vi "grabber_raps.vi"() -> ()   [LabVIEW 2010]
uses:
  command_enum.ctl
  status_enum.ctl
  FPGAWrapperMH120124RAPS_PXI7813R/settings_cluster_raps.ctl
  common_typedefs/channels_cluster.ctl
  fpgaVIsAndControls/gate_cluster.ctl
  common_typedefs/gate_parameters_cluster.ctl
  motion_correction_cluster.ctl
  gui_refs.ctl
  <vilib>/rvi/interface/nirviReadWriteControl/nirviReadWriteControl.xnode
  FPGA_raps_reference.ctl
  <vilib>/rvi/interface/common/niFpgaNodeNameForErrorReporting.ctl
  <vilib>/rvi/errors/niLvFpgaWhatHappensToTopLevelVI.ctl
  <vilib>/dex/Flush And Wait Empty Condition.ctl
  <vilib>/rvi/interface/nirviMethod/nirviMethod.xnode
  <vilib>/rvi/interface/nirviCloseFPGA/nirviCloseFPGA.xnode
  <vilib>/Utility/error.llb/Error Cluster From Error Code.vi
  <vilib>/rvi/errors/niLvFpgaAdjustHostInterfaceError.vi
  <vilib>/FPGAPlugInAG/Dynamic/niLvFpga_Close_Dynamic.vi
  NiFpgaLv.dll
panel:
  out "offset (y,x)":i16[](array[numeric])
  in  "total amount pixels":i32
  in  "channel":i8
  in  "# square points":i32
  in  "reference array":u16[][](graph)
  out "data out":T1={"number of pixels"=0, "point package size"=0, "maximum bit-depth"=0, "AOD amplitude"=0, "pixel dwell time"=0.0, "ra trajectory pixels (data/pixels transfered)"=0, "channel offsets"={"channel 0"=0, "channel 1"=0, "channel 2"=0, "channel 3"=0}, "offset (Hz)"=[], "RAPS array"=[], "gates"=[], "enable clocks?"=-1, "motion correction"={"reference array"=[], "# square points"=0, "channel"=0}}
  in  "first pixel is zero?":bool caption="first pixel is zero? (set to TRUE for debugging only)"
  out "current pixel no.":i64
  out "read size":u32
  out "Elements Remaining":u32
  out "stop":bool
  out "current status":T5
  out "pixel no.":i64
  out "last command_not_acq":T6
  out "FIFO overflow?":bool
  out "last command?":T6
  out "error out":errorcluster
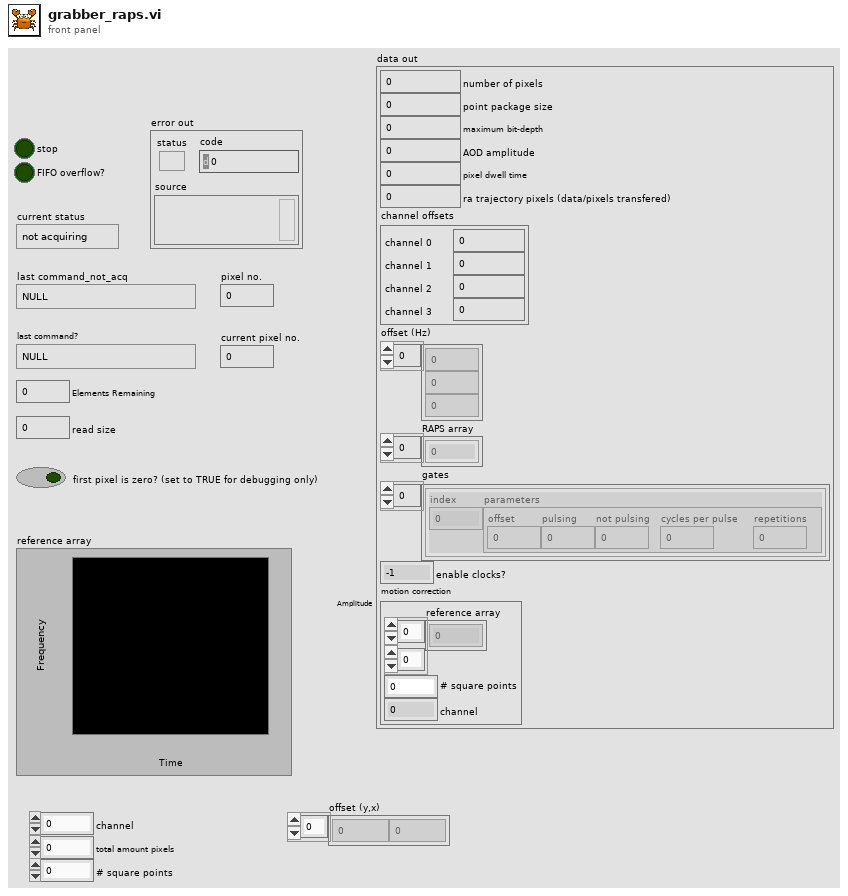
[diagram p1: front panel]
types:
  T1 = typedef "settings_cluster_raps.ctl" = cluster{"number of pixels":i64, "point package size":u8, "maximum bit-depth":i8, "AOD amplitude":u16, "pixel dwell time":dbl, "ra trajectory pixels (data/pixels transfered)":u32, "channel offsets":T2, "offset (Hz)":dbl[], "RAPS array":u64[], "gates":T3[], "enable clocks?":i16, "motion correction":cluster{"reference array":u16[][], "# square points":i32, "channel":i8}}
  T2 = typedef "channels_cluster.ctl" = cluster{"channel 0":u32, "channel 1":u32, "channel 2":u32, "channel 3":u32}
  T3 = typedef "gate_cluster.ctl" = cluster{"index":i32, "parameters":T4}
  T4 = typedef "gate_parameters_cluster.ctl" = cluster{"offset":i64, "pulsing":i64, "not pulsing":i64, "cycles per pulse":i64, "repetitions":i64}
  T5 = typedef "status_enum.ctl" = enum16{"not acquiring", "acquiring"}
  T6 = typedef "command_enum.ctl" = enum8{"NULL", "update", "start", "stop", "reset", "shut-down"}
  T7 = typedef "gui_refs.ctl" = cluster{"reference array":refnum<vi>, "total amount pixels":refnum<vi>, "# square points":refnum<vi>, "channel":refnum<vi>}
  T8 = typedef "motion_correction_cluster.ctl" = cluster{"reception":cluster{"square length":i32, "offset":i32, "# squares out":i32, "left over":u16[], "raps points length":i32}, "fft":cluster{"reference":dbl[][]}}
  T9 = typedef "FPGA_raps_reference.ctl" = refnum<k20>
  T10 = typedef "network_streaming_queues_cluster.ctl" = cluster{"command reader":refnum<k21>, "data writer":refnum<k21>, "raps reader":refnum<k21>, "settings framescan reader":refnum<k21>, "configuration framescan reader":refnum<k21>, "settings raps reader":refnum<k21>, "configuration raps reader":refnum<k21>, "update queue":refnum<queue>}
  T11 = typedef "niFpgaNodeNameForErrorReporting.ctl" = enum16{"Open FPGA VI Reference", "Read/Write Control", "Invoke Method: Abort", "Invoke Method: Acknowledge IRQ", "Invoke Method: Download", "Invoke Method: FIFO.Configure", "Invoke Method: FIFO.Read", "Invoke Method: FIFO.Start", "Invoke Method: FIFO.Stop", "Invoke Method: FIFO.Write", "Invoke Method: Reset", "Invoke Method: Run", "Invoke Method: Wait on IRQ", "Close FPGA VI Reference"}
  T12 = typedef "niLvFpgaWhatHappensToTopLevelVI.ctl" = enum16{"top level VI scripted behind XNode", "top level VI inlined behind XNode"}
  T13 = typedef "Flush And Wait Empty Condition.ctl" = u8
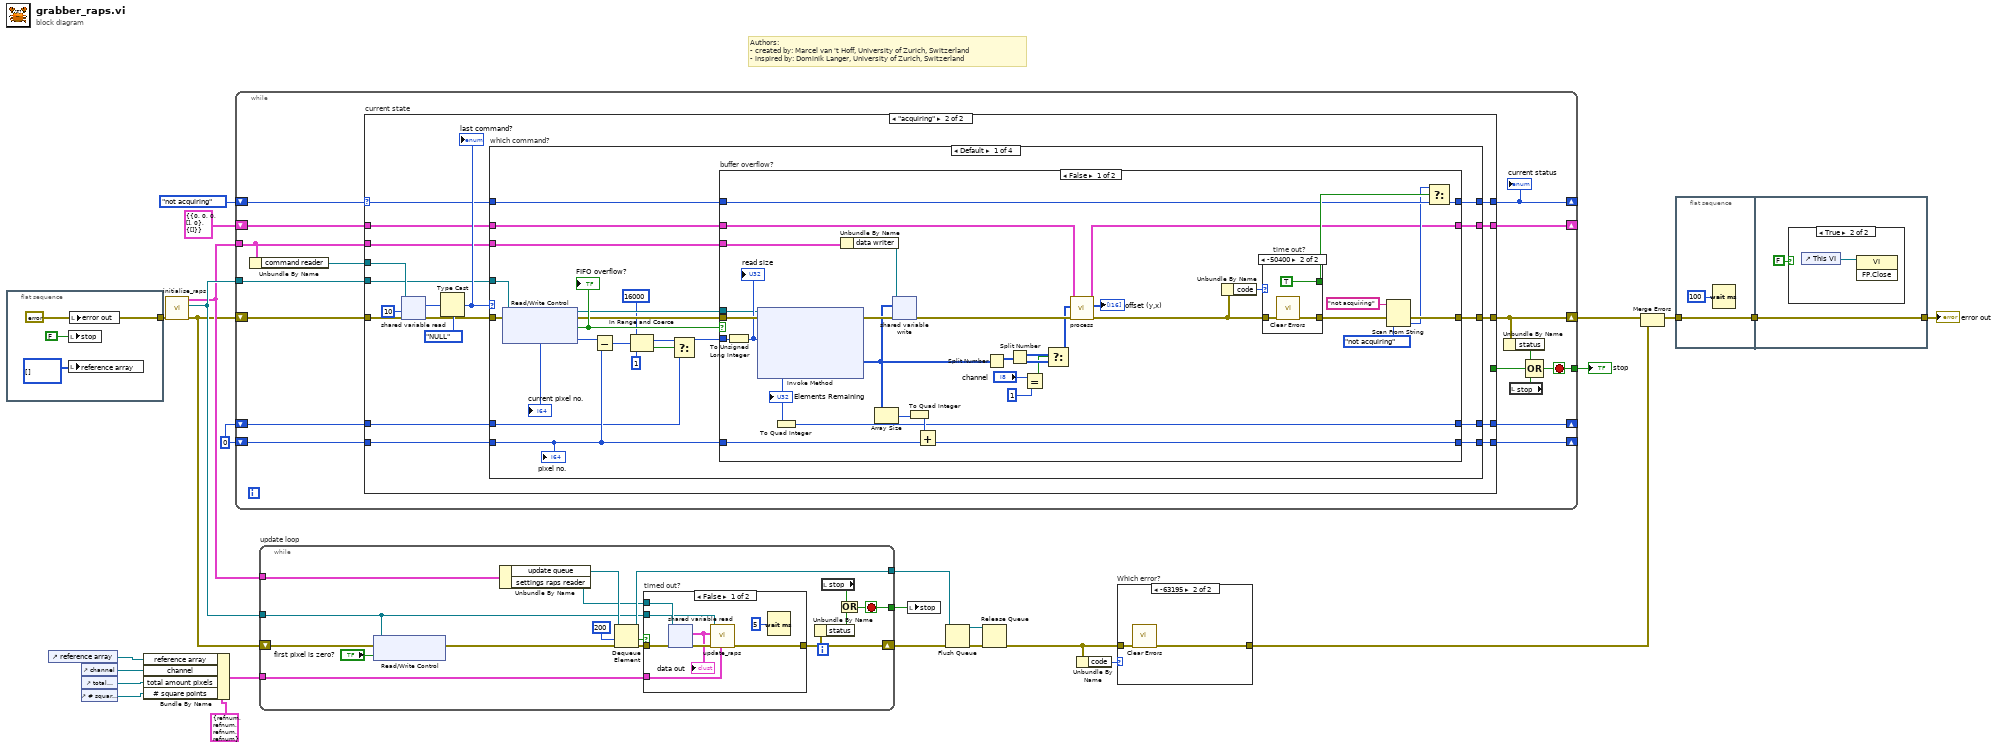
[diagram p0: block diagram]
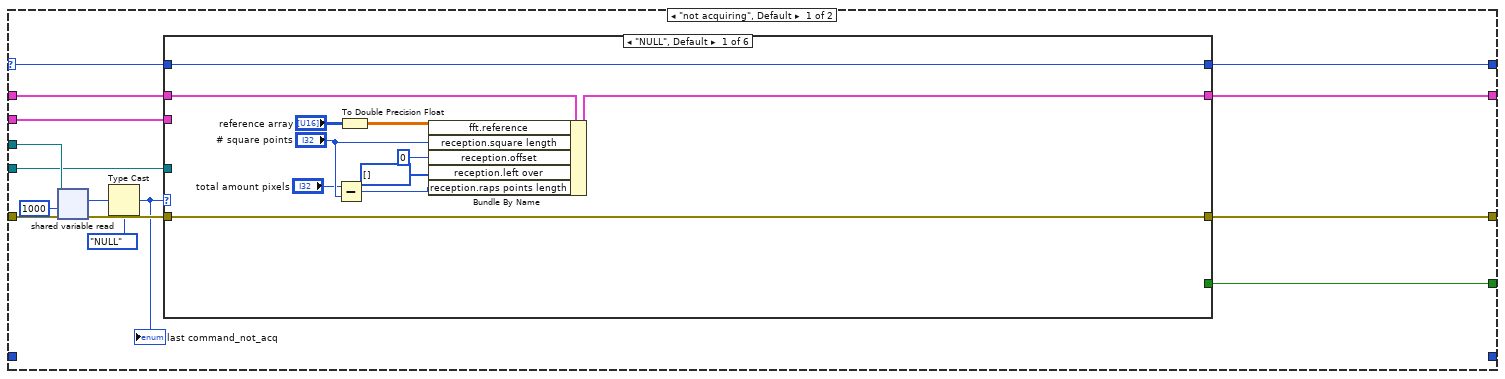
[diagram p5: hidden frame]
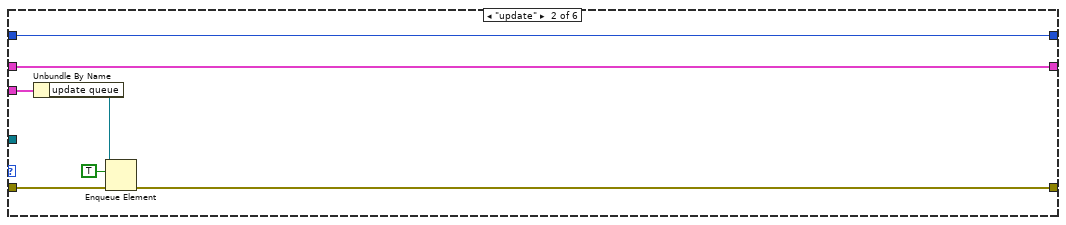
[diagram p6: hidden frame]
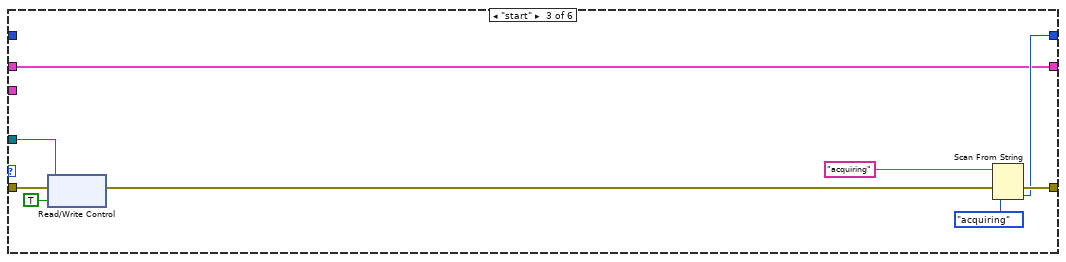
[diagram p7: hidden frame]
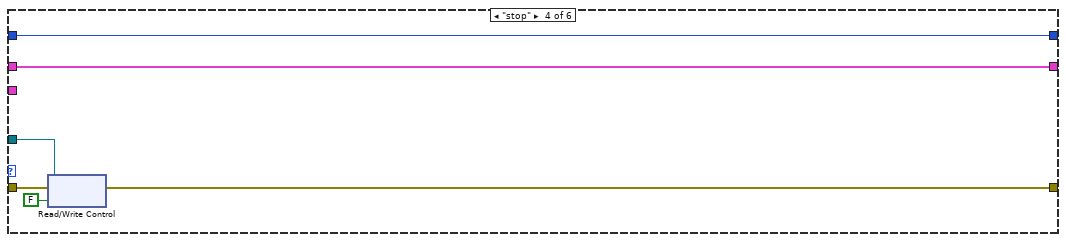
[diagram p8: hidden frame]
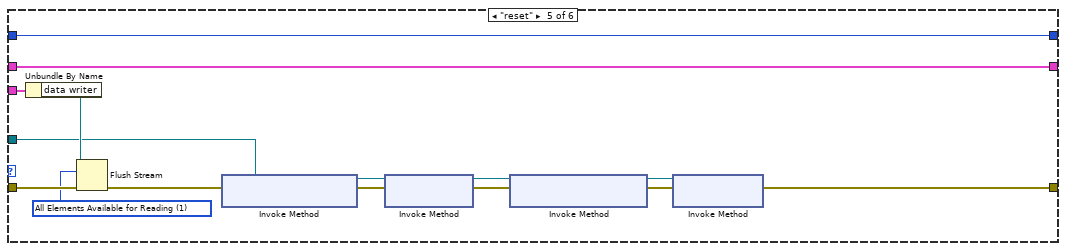
[diagram p9: hidden frame]
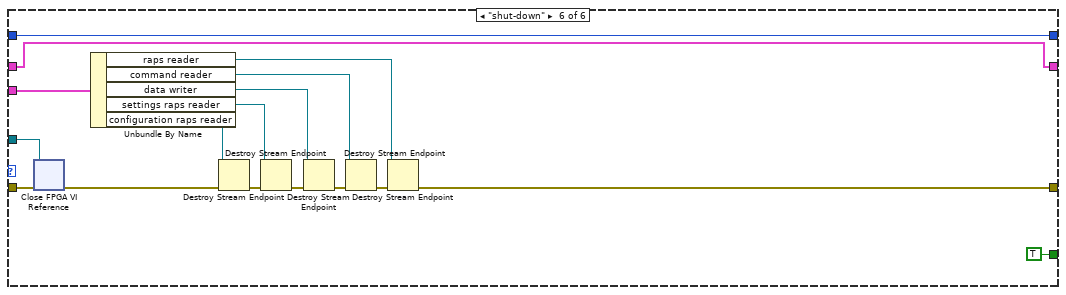
[diagram p10: hidden frame]
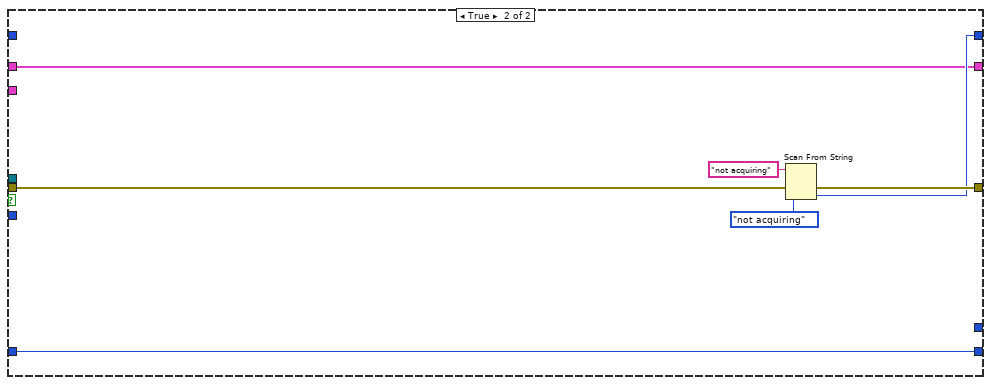
[diagram p12: hidden frame]
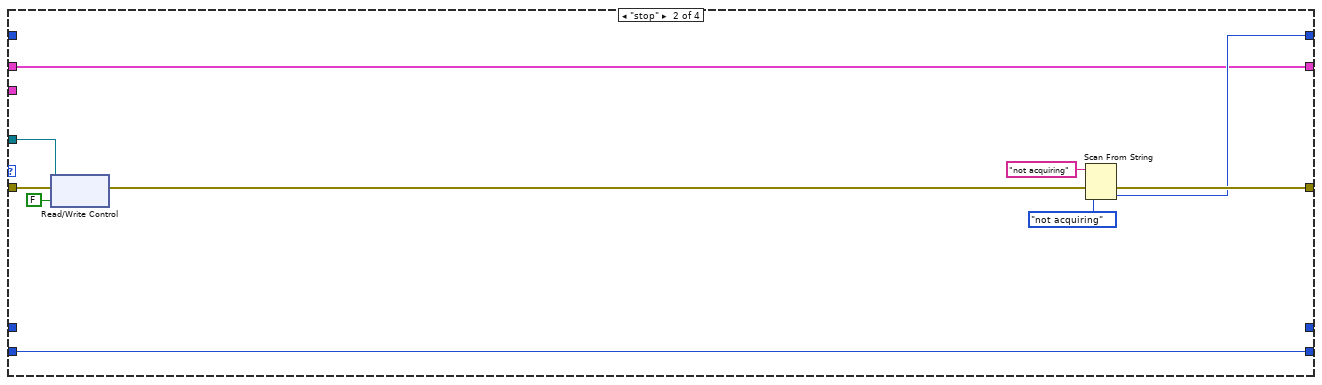
[diagram p13: hidden frame]
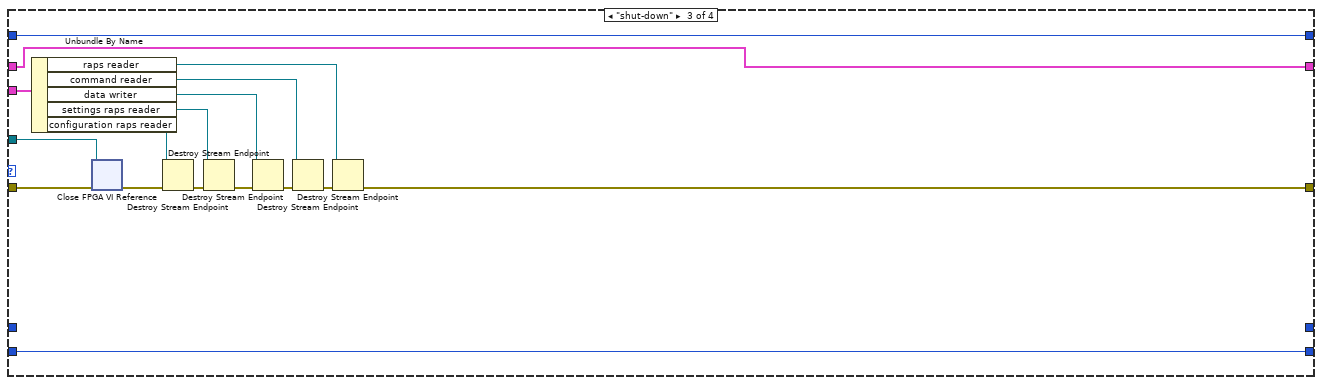
[diagram p14: hidden frame]
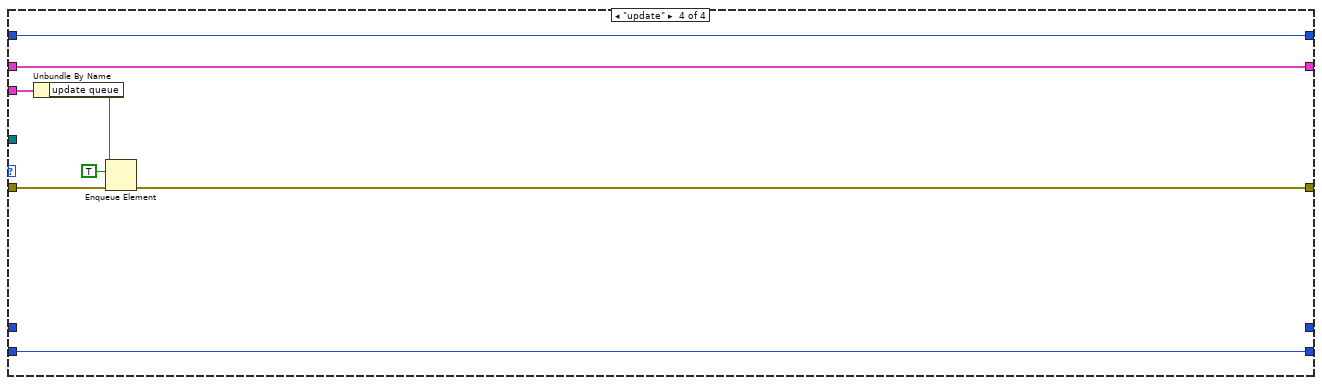
[diagram p15: hidden frame]
diagram:
  w13 = i64 0
  # "Authors:\n- created by: Marcel van 't Hoff, University of Zurich, Switzerland\n- inspired by: Dominik Langer, University of Zurich, Switzerland"
  n1 = flat-sequence {
    tunnel: [w29] -> w14
    frame #0 {
      w29 = errorcluster {"status"=FALSE, "code"=0, "source"=""} ("error in (no error)")
      n2 = local write "stop"(FALSE ("stop")) -> ()
      n3 = local write "reference array"(u16[][] [] ("reference array")) -> ()
      n4 = local write "error out"(w29) -> ()
    }
  }
  n5 = control-ref of="reference array"() -> (w5:refnum<vi>)
  n6 = control-ref of="channel"() -> (w1:refnum<vi>)
  n7 = control-ref of="total amount pixels"() -> (w3:refnum<vi>)
  n8 = control-ref of="# square points"() -> (w4:refnum<vi>)
  n9 = Bundle By Name(cluster=T7 {"reference array"=refnum, "total amount pixels"=refnum, "# square points"=refnum, "channel"=refnum} ("gui refs"), "reference array"=w5, "channel"=w1, "total amount pixels"=w3, "# square points"=w4) -> (w2:T7)
  n10 = call "initialise_raps.vi"("error in (no error)"=w14) -> ("error out"=w12:errorcluster, "FPGA VI Reference"=w25:T9, "network streaming queues out"=w24:T10)  [unwired: 8 in]
  n11 = while {
    tunnel: w25 -> [w43]
    tunnel: w24 -> [w44]
    shift-right: [w39] -> _
    shift-left: status_enum."not acquiring" ("status enum") -> [w46]
    shift-right: [w38] -> w19
    shift-left: w12 -> [w42]
    shift-right: [w40] -> _
    shift-left: w13 -> [w41]
    tunnel: [w35] -> w18
    shift-right: [w34] -> _
    shift-left: w13 -> [w33]
    shift-right: [w30] -> _
    shift-left: T8 {"reception"={"square length"=0, "offset"=0, "# squares out"=0, "left over"=[], "raps points length"=0}, "fft"={"reference"=[]}} ("cluster out") -> [w31]
    stop <- w35 stop-if-true
    n12 = Unbundle By Name(w44) -> ("command reader"=w45:refnum<k21>)
    n13 = case "current state" shown="\"acquiring\"" w46 {
      selector: w46 -> [w55 w310]
      tunnel: w45 -> [w60 w316]
      tunnel: w44 -> [w57 w311]
      tunnel: w43 -> [w58 w309]
      tunnel: w42 -> [w61 w315]
      tunnel: w41 -> [_ w308]
      tunnel: [_ w307] -> w40
      tunnel: [w54 w306] -> w38
      tunnel: [w56 w305] -> w39
      tunnel: [w53 _] -> w36
      tunnel: [_ w302] -> w34
      tunnel: w33 -> [_ w301]
      tunnel: w31 -> [w48 w300]
      tunnel: [w47 w299] -> w30
      frame "not acquiring", Default {
        n14 = shared-variable-read(w60, w61, 1000 ("timeout in ms (-1)")) -> (w59:errorcluster, w50:u8)  [unwired: 2 out]
        n15 = Type Cast(type=command_enum."NULL" ("command"), x=w50) -> (*(type *) &x=w51:T6)
        "last command_not_acq" <- w51
        n16 = case shown="\"NULL\", Default" w51 {
          tunnel: w59 -> [w71 w75 w88 w132 w187 w292]
          tunnel: w58 -> [_ _ w87 w133 w177 w291]
          tunnel: w57 -> [_ w76 _ _ w186 w281]
          tunnel: [w72 w79 w82 w130 w185 w289] -> w56
          tunnel: w55 -> [w72 w79 _ w130 w185 w289]
          tunnel: [w71 w74 w85 w131 w180 w278] -> w54
          tunnel: [_ _ _ _ _ TRUE] -> w53
          tunnel: [w68 w73 w80 w128 w173 w276] -> w47
          tunnel: w48 -> [w69 w73 w80 w128 w173 w276]
          frame "NULL", Default {
            n17 = Subtract(x="total amount pixels", y="# square points") -> (x-y=w62:i32)
            n18 = To Double Precision Float(number="reference array") -> (double precision float=w67:dbl[][])
            n19 = Bundle By Name(cluster=w69, "fft.reference"=w67, "reception.square length"="# square points", "reception.offset"=0, "reception.left over"=u16[] [], "reception.raps points length"=w62) -> (w68:T8)
          }
          frame "update" {
            n20 = Unbundle By Name(w76) -> ("update queue"=w77:refnum<queue>)
            n21 = Enqueue Element(queue=w77, element=TRUE, error in (no error)=w75) -> (error out=w74:errorcluster)  [unwired: 1 in, 2 out]
          }
          frame "start" {
            n22 = xnode "Read/Write Control"("FPGA VI Reference In"=w87, "error in"=w88, "acquire?"=TRUE) -> ("error out"=w86:errorcluster)  [unwired: 1 out]
            n23 = Scan From String(input string="acquiring", error in=w86, default 1=status_enum."acquiring" ("status enum")) -> (error out=w85:errorcluster, output 1=w82:T5)  [unwired: 2 in, 2 out]
          }
          frame "stop" {
            n24 = xnode "Read/Write Control"("FPGA VI Reference In"=w133, "error in"=w132, "acquire?"=FALSE) -> ("error out"=w131:errorcluster)  [unwired: 1 out]
          }
          frame "reset" {
            w178 = T13 1 items=["All Elements Read From Stream", "All Elements Available for Reading"] ("wait condition")
            n25 = Unbundle By Name(w186) -> ("data writer"=w179:refnum<k21>)
            n26 = Flush Stream(8:w187, 10:w178, 11:w179) -> (0:w176:errorcluster)  [unwired: 1 in, 2 out]
            n27 = xnode "Invoke Method"("FPGA VI Reference In"=w177, "error in"=w176) -> ("FPGA VI Reference Out"=w184:T9, "error out"=w183:errorcluster)
            n28 = xnode "Invoke Method"("FPGA VI Reference In"=w184, "error in"=w183) -> ("FPGA VI Reference Out"=w174:T9, "error out"=w175:errorcluster)
            n29 = xnode "Invoke Method"("FPGA VI Reference In"=w174, "error in"=w175) -> ("FPGA VI Reference Out"=w182:T9, "error out"=w181:errorcluster)
            n30 = xnode "Invoke Method"("FPGA VI Reference In"=w182, "error in"=w181) -> ("error out"=w180:errorcluster)  [unwired: 1 out]
          }
          frame "shut-down" {
            n31 = xnode "Close FPGA VI Reference"("FPGA VI Reference In"=w291, "error in"=w292) -> ("error out"=w279:errorcluster)
            n32 = Unbundle By Name(w281) -> ("raps reader"=w282:refnum<k21>, "command reader"=w284:refnum<k21>, "data writer"=w285:refnum<k21>, "settings raps reader"=w288:refnum<k21>, "configuration raps reader"=w280:refnum<k21>)
            n33 = Destroy Stream Endpoint(8:w279, 11:w280) -> (0:w286:errorcluster)
            n34 = Destroy Stream Endpoint(8:w286, 11:w288) -> (0:w277:errorcluster)
            n35 = Destroy Stream Endpoint(8:w277, 11:w285) -> (0:w287:errorcluster)
            n36 = Destroy Stream Endpoint(8:w287, 11:w284) -> (0:w283:errorcluster)
            n37 = Destroy Stream Endpoint(8:w283, 11:w282) -> (0:w278:errorcluster)
          }
        }
      }
      frame "acquiring" {
        n38 = shared-variable-read(w316, w315, 10 ("timeout in ms (-1)")) -> (w312:errorcluster, w304:u8)  [unwired: 2 out]
        n39 = Type Cast(type=command_enum."NULL" ("command"), x=w304) -> (*(type *) &x=w313:T6)
        "last command?" <- w313
        n40 = case "which command?" shown="Default" w313 {
          tunnel: w312 -> [w337 w543 w594 w609]
          tunnel: w311 -> [w333 _ w592 w607]
          tunnel: w310 -> [w329 _ w585 w612]
          tunnel: w309 -> [w338 w542 w593 _]
          tunnel: w308 -> [w331 w541 w586 w613]
          tunnel: [w332 w541 w586 w613] -> w307
          tunnel: [w330 w537 w587 w608] -> w306
          tunnel: [w328 w536 w585 w612] -> w305
          tunnel: [w324 _ _ _] -> w302
          tunnel: w301 -> [w321 _ _ _]
          tunnel: w300 -> [w318 w534 w583 w606]
          tunnel: [w317 w534 w583 w606] -> w299
          frame Default {
            n41 = xnode "Read/Write Control"("FPGA VI Reference In"=w338, "error in"=w337) -> ("FPGA VI Reference Out"=w335:T9, "error out"=w334:errorcluster, "FIFO_DMA0 full?"=w336:bool, "current pixel no."=w319:i64)
            "FIFO overflow?" <- w336
            "current pixel no." <- w319
            n42 = Subtract(x=w319, y=w331) -> (x-y=w327:i64)
            n43 = In Range and Coerce(upper limit=i64 16000, x=w327, lower limit=i64 1) -> (coerced(x)=w322:i64, In Range?=w323:bool)
            n44 = Select(t=w322, s=w323, f=w321) -> (s? t:f=w320:i64)
            n45 = case "buffer overflow?" shown="False" w336 {
              tunnel: w320 -> [w373 _]
              tunnel: w335 -> [w360 _]
              tunnel: w334 -> [w370 w455]
              tunnel: w333 -> [w372 _]
              tunnel: [w367 w457] -> w332
              tunnel: w331 -> [w366 w457]
              tunnel: [w355 w454] -> w330
              tunnel: w329 -> [w363 _]
              tunnel: [w362 w452] -> w328
              tunnel: [w358 _] -> w324
              tunnel: w318 -> [w343 w451]
              tunnel: [w344 w451] -> w317
              frame False {
                n46 = To Unsigned Long Integer(number=w373) -> (unsigned 32bit integer=w361:u32)
                "read size" <- w361
                n47 = xnode "Invoke Method"("FPGA VI Reference In"=w360, "error in"=w370, "Number of Elements"=w361) -> ("error out"=w352:errorcluster, "Data"=w351:u64[], "Elements Remaining"=w359:u32)  [unwired: 1 in, 1 out]
                "Elements Remaining" <- w359
                n48 = To Quad Integer(1:w359) -> (0:w358:i64)
                n49 = Unbundle By Name(w372) -> ("data writer"=w371:refnum<k21>)
                n50 = Array Size(array=w351) -> (size(s)=w369:i32)
                n51 = shared-variable-write(w371, w352, w351) -> (w342:errorcluster)  [unwired: 1 in, 2 out]
                n52 = To Quad Integer(1:w369) -> (0:w368:i64)
                n53 = Add(x=w368, y=w366) -> (x+y=w367:i64)
                n54 = Split Number(x=w351) -> (hi(x)=w350:u32[])  [unwired: 1 out]
                n55 = Split Number(x=w350) -> (hi(x)=w349:u16[], lo(x)=w348:u16[])
                n56 = Equal?(x="channel", y=i8 1) -> (x = y?=w345:bool)
                n57 = Select(t=w349, s=w345, f=w348) -> (s? t:f=w340:u16[])
                n58 = call "process.vi"("error in (no error)"=w342, "array in"=w340, "cluster in"=w343) -> ("error out"=w341:errorcluster, "offset"=→"offset (y,x)":i16[], "cluster out"=w344:T8)  [unwired: 6 in]
                n59 = Unbundle By Name(w341) -> ("code"=w365:i32)
                n60 = case "time out?" shown="-50400" w365 {
                  tunnel: w341 -> [w374 w377]
                  tunnel: [w374 w376] -> w354
                  tunnel: [_ TRUE] -> w364
                  frame Default {
                  }
                  frame -50400 {
                    n61 = call <vilib>:"Clear Errors.vi"("error in (no error)"=w377) -> ("error out"=w376:errorcluster)  [unwired: 6 in]
                  }
                }
                n62 = Scan From String(input string="not acquiring", error in=w354, default 1=status_enum."not acquiring" ("status enum")) -> (error out=w355:errorcluster, output 1=w353:T5)  [unwired: 2 in, 2 out]
                n63 = Select(t=w353, s=w364, f=w363) -> (s? t:f=w362:T5)
              }
              frame True {
                n64 = Scan From String(input string="not acquiring", error in=w455, default 1=status_enum."not acquiring" ("status enum")) -> (error out=w454:errorcluster, output 1=w452:T5)  [unwired: 2 in, 2 out]
              }
            }
            "pixel no." <- w331
          }
          frame "stop" {
            n65 = xnode "Read/Write Control"("FPGA VI Reference In"=w542, "error in"=w543, "acquire?"=FALSE) -> ("error out"=w538:errorcluster)  [unwired: 1 out]
            n66 = Scan From String(input string="not acquiring", error in=w538, default 1=status_enum."not acquiring" ("status enum")) -> (error out=w537:errorcluster, output 1=w536:T5)  [unwired: 2 in, 2 out]
          }
          frame "shut-down" {
            n67 = Unbundle By Name(w592) -> ("raps reader"=w588:refnum<k21>, "command reader"=w590:refnum<k21>, "data writer"=w591:refnum<k21>, "settings raps reader"=w599:refnum<k21>, "configuration raps reader"=w598:refnum<k21>)
            n68 = xnode "Close FPGA VI Reference"("FPGA VI Reference In"=w593, "error in"=w594) -> ("error out"=w597:errorcluster)
            n69 = Destroy Stream Endpoint(8:w597, 11:w598) -> (0:w595:errorcluster)
            n70 = Destroy Stream Endpoint(8:w595, 11:w599) -> (0:w584:errorcluster)
            n71 = Destroy Stream Endpoint(8:w584, 11:w591) -> (0:w596:errorcluster)
            n72 = Destroy Stream Endpoint(8:w596, 11:w590) -> (0:w589:errorcluster)
            n73 = Destroy Stream Endpoint(8:w589, 11:w588) -> (0:w587:errorcluster)
          }
          frame "update" {
            n74 = Unbundle By Name(w607) -> ("update queue"=w610:refnum<queue>)
            n75 = Enqueue Element(queue=w610, element=TRUE, error in (no error)=w609) -> (error out=w608:errorcluster)  [unwired: 1 in, 2 out]
          }
        }
      }
    }
    "current status" <- w39
    n76 = Unbundle By Name(w38) -> ("status"=w37:bool)
    n77 = local read "stop"() -> (w32:bool)
    n78 = Compound Arithmetic op=OR(w37, w36, w32) -> (w35:bool)
  }
  "stop" <- w18
  n79 = while "update loop" {
    tunnel: w25 -> [w619]
    tunnel: w24 -> [w629]
    tunnel: [w624] -> w20
    shift-right: [w628] -> w21
    shift-left: w12 -> [w618]
    tunnel: [w615] -> w11
    tunnel: w2 -> [w614]
    stop <- w615 stop-if-true
    n80 = xnode "Read/Write Control"("FPGA VI Reference In"=w619, "error in"=w618, "first pixel black?"="first pixel is zero?") -> ("error out"=w617:errorcluster)  [unwired: 1 out]
    n81 = Unbundle By Name(w629) -> ("update queue"=w625:refnum<queue>, "settings raps reader"=w623:refnum<k21>)
    n82 = Dequeue Element(queue=w625, timeout in ms (-1)=200, error in (no error)=w617) -> (queue out=w624:refnum<queue>, timed out?=w620:bool, error out=w621:errorcluster)  [unwired: 1 out]
    n83 = case "timed out?" shown="False" w620 {
      tunnel: w623 -> [w676 _]
      tunnel: w619 -> [w674 _]
      tunnel: [w673 w677] -> w628
      tunnel: w621 -> [w671 w677]
      tunnel: w614 -> [w669 _]
      frame False {
        n84 = shared-variable-read(w676, w671) -> (w675:errorcluster, w670:T1)  [unwired: 1 in, 2 out]
        "data out" <- w670
        n85 = call "update_raps.vi"("gui refs"=w669, "error in (no error)"=w675, "settings cluster"=w670, "FPGA VI Reference In"=w674) -> ("error out"=w673:errorcluster)  [unwired: 7 in]
        n86 = Wait (ms)(milliseconds to wait=u32 5) -> ()  [unwired: 1 out]
      }
      frame True {
      }
    }
    n87 = Unbundle By Name(w628) -> ("status"=w627:bool)
    n88 = local read "stop"() -> (w626:bool)
    n89 = Or(x=w626, y=w627) -> (x .or. y?=w615:bool)
  }
  n90 = local write "stop"(w11) -> ()
  n91 = Flush Queue(queue=w20, error in (no error)=w21) -> (queue out=w22:refnum<queue>, error out=w23:errorcluster)  [unwired: 1 out]
  n92 = Release Queue(queue=w22, error in (no error)=w23) -> (error out=w9:errorcluster)  [unwired: 1 in, 2 out]
  n93 = Unbundle By Name(w9) -> ("code"=w10:i32)
  n94 = case "Which error?" shown="-63195" w10 {
    tunnel: w9 -> [w678 w680]
    tunnel: [w678 w679] -> w8
    frame Default {
    }
    frame -63195 {
      n95 = call <vilib>:"Clear Errors.vi"("error in (no error)"=w680) -> ("error out"=w679:errorcluster)  [unwired: 6 in]
    }
  }
  n96 = Merge Errors(w19, w8) -> (w16:errorcluster)
  n97 = flat-sequence {
    tunnel: w16 -> [w682]
    tunnel: [w682] -> w17
    tunnel: [w684] -> w15
    tunnel: w17 -> [w684]
    frame #0 {
      n98 = Wait (ms)(milliseconds to wait=u32 100) -> ()  [unwired: 1 out]
    }
    frame #1 {
      n99 = case shown="True" FALSE {
        frame False {
        }
        frame True {
          n100 = control-ref of="This VI"() -> (w685:refnum<vi>)
          n101 = invoke class="VI" method="FP.Close"(reference=w685) -> ()  [unwired: 2 in, 3 out]
        }
      }
    }
  }
  "error out" <- w15
